vi "5 - filtering.vi"() -> ()   [LabVIEW 2025]
uses:
  <vilib>/Analysis/3filter.llb/Butterworth Filter (DBL).vi
  <vilib>/Waveform/WDTFileIO.llb/Export Waveform To Spreadsheet File.vi
  <vilib>/measure/NI_MABase.lvlib
  <vilib>/Analysis/NI_AALBase.lvlib
panel:
  in  "Sampling info":T1={"frequency [Hz]"=1000.0, "number of samples"=1000.0} {"number of samples" format="%.2p"; "frequency [Hz]" format="%.2p"}
  in  "time to refresh [ms]":u32
  in  "off/on":bool
  in  "off/on":bool
  in  "off/ on":bool
  out "filter characteristic":u16(ring) items=["Butterworth Filter", "Chebyshev Filter", "Elliptic Filter", "Bessel Filter"]
  in  "Tab Control":enum32{"waveform", "noise"}(tab)
  in  "phase [deg]":dbl(slide) scale=0.0..360.0
  in  "frequency [Hz]":dbl=10.0 min=0.0 format="%.0p"
  in  "offset [V]":dbl(slide) scale=0.0..10.0
  in  "amplitude [V]":dbl=1.0 min=0.0 format="%.0p"
  in  "signal type":u16(ring) items=["sine wave", "triangle wave", "square wave", "sawtooth wave"]
  in  "standard deviation":dbl=1.0 min=0.0 max=100.0 step=1.0 format="%.2f"
  in  "Tab Control":enum32{"waveform", "noise"}(tab)
  in  "frequency [Hz]":dbl=10.0 min=0.0 format="%.0p"
  in  "phase [deg]":dbl(slide) scale=0.0..360.0
  in  "offset [V]":dbl(slide) scale=0.0..10.0
  in  "amplitude [V]":dbl=1.0 min=0.0 format="%.0p"
  in  "signal type 2":u16(ring) items=["sine wave", "triangle wave", "square wave", "sawtooth wave"]
  in  "standard deviation":dbl=1.0 min=0.0 max=100.0 step=1.0 format="%.2f"
  in  "Tab Control":enum32{"waveform", "noise"}(tab)
  in  "phase [deg]":dbl(slide) scale=0.0..360.0
  in  "frequency [Hz]":dbl=10.0 min=0.0 format="%.0p"
  in  "offset [V]":dbl(slide) scale=0.0..10.0
  in  "amplitude [V]":dbl=1.0 min=0.0 format="%.0p"
  in  "signal type":u16(ring) items=["sine wave", "triangle wave", "square wave", "sawtooth wave"]
  in  "standard deviation":dbl=1.0 min=0.0 max=100.0 step=1.0 format="%.2f"
  in  "Tab Control":enum32{"Page 2"}(tab)
  in  "order":i32=2 min=0
  in  "high cutoff freq [Hz]":dbl=0.45000000000000007 min=0.0 format="%.1f"
  in  "filter type":u16(ring) items=["lowpass", "highpass", "bandpass", "bandstop"]
  in  "init/cont":bool
  in  "low cutoff freq [Hz]":dbl=0.12500000000000006 min=0.0 format="%.1f"
  out "Filter output":cluster{i32, dbl, "Filtered X":dbl[]}(graph)
  out "Filter input":waveform(dbl)(graph)
  in  "stop":bool
  # "Channel A"
  # "Channel B"
  # "Channel C"
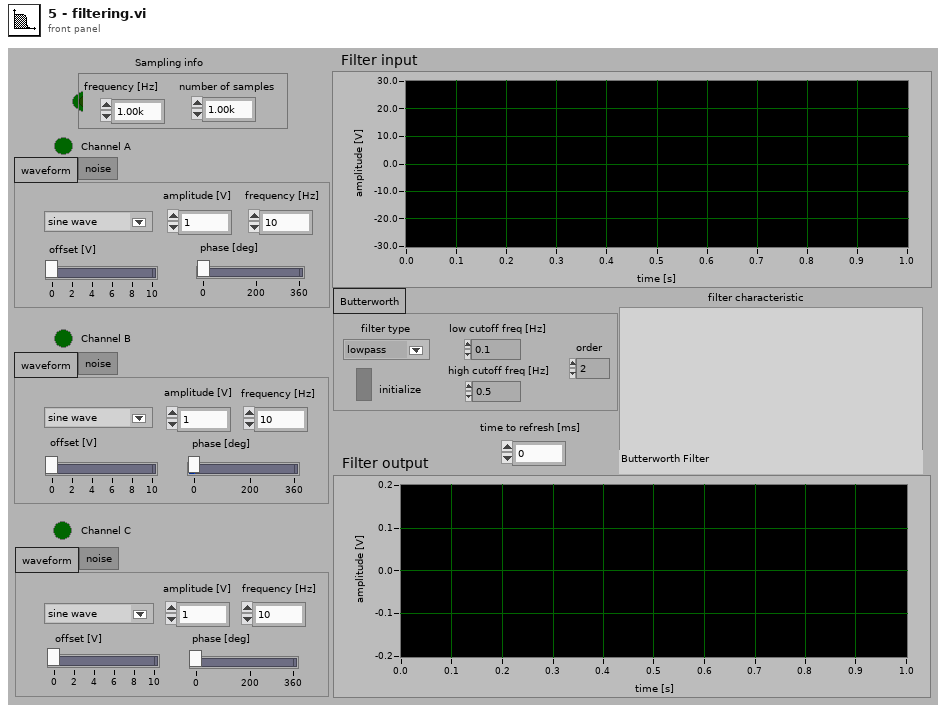
[diagram p1: front panel]
types:
  T1 = cluster{"frequency [Hz]":dbl, "number of samples":dbl}
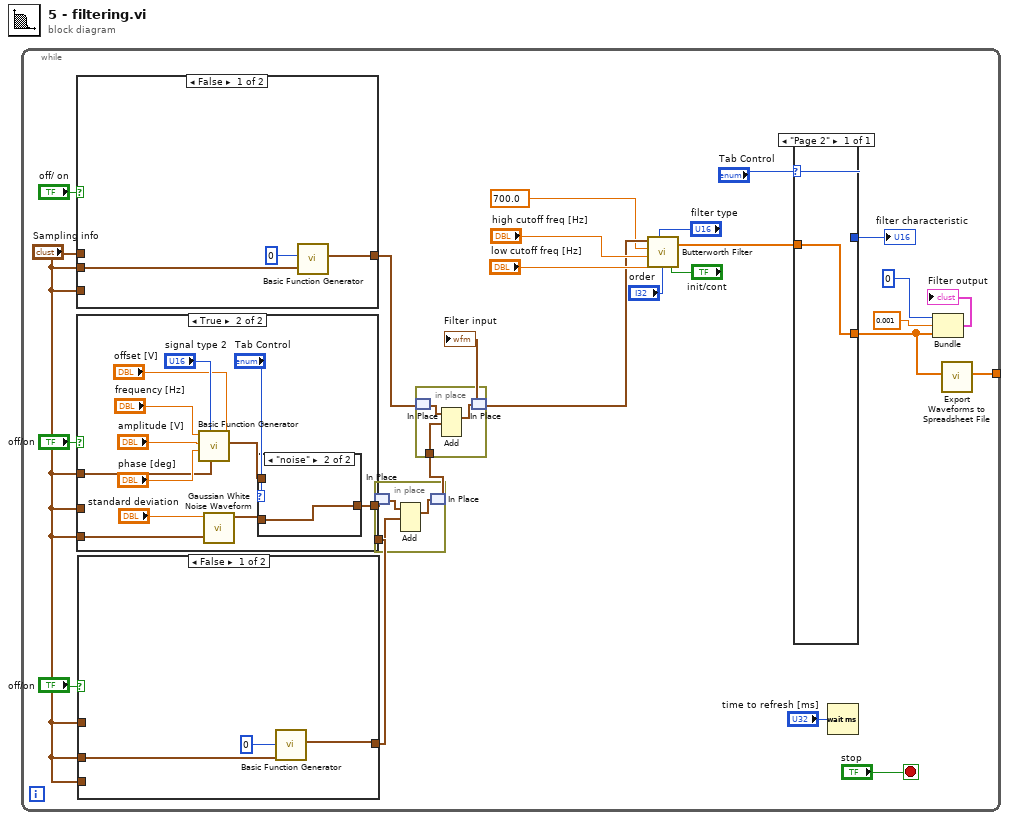
[diagram p0: block diagram]
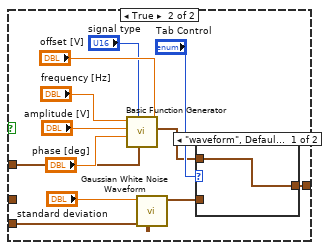
[diagram p2: hidden frame]
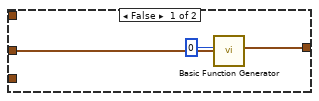
[diagram p4: hidden frame]
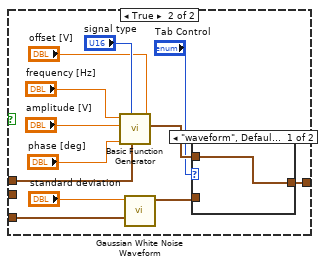
[diagram p6: hidden frame]
diagram:
  n1 = while {
    tunnel: [w6] -> w1
    stop <- "stop" stop-if-true
    n2 = case shown="False" "off/ on" {
      tunnel: [w68 w72] -> w5
      tunnel: "Sampling info" -> [_ w70]
      tunnel: "Sampling info" -> [_ w69]
      tunnel: "Sampling info" -> [w66 _]
      frame False {
        n3 = call <vilib>:"Basic Function Generator.vi"("sampling info"=w66, "amplitude"=0) -> ("signal out"=w68:waveform(dbl))  [unwired: 7 in, 2 out]
      }
      frame True {
        n4 = call <vilib>:"Basic Function Generator.vi"("offset"="offset [V]", "sampling info"=w69, "signal type"="signal type", "phase"="phase [deg]", "amplitude"="amplitude [V]", "frequency"="frequency [Hz]") -> ("signal out"=w80:waveform(dbl))  [unwired: 3 in, 2 out]
        n5 = call <vilib>:"Gaussian White Noise Waveform.vi"("sampling info"=w70, "standard deviation"="standard deviation") -> ("signal out"=w74:waveform(dbl))  [unwired: 3 in, 6 out]
        n6 = case shown="\"waveform\", Default" "Tab Control" {
          tunnel: w80 -> [w81 _]
          tunnel: w74 -> [_ w82]
          tunnel: [w81 w82] -> w72
          frame "waveform", Default {
          }
          frame "noise" {
          }
        }
      }
    }
    n7 = case shown="True" "off/on" {
      tunnel: [w50 w54] -> w21
      tunnel: "Sampling info" -> [_ w53]
      tunnel: "Sampling info" -> [_ w52]
      tunnel: "Sampling info" -> [w49 _]
      frame False {
        n8 = call <vilib>:"Basic Function Generator.vi"("sampling info"=w49, "amplitude"=0) -> ("signal out"=w50:waveform(dbl))  [unwired: 7 in, 2 out]
      }
      frame True {
        n9 = call <vilib>:"Basic Function Generator.vi"("offset"="offset [V]", "sampling info"=w52, "signal type"="signal type 2", "phase"="phase [deg]", "amplitude"="amplitude [V]", "frequency"="frequency [Hz]") -> ("signal out"=w63:waveform(dbl))  [unwired: 3 in, 2 out]
        n10 = call <vilib>:"Gaussian White Noise Waveform.vi"("sampling info"=w53, "standard deviation"="standard deviation") -> ("signal out"=w62:waveform(dbl))  [unwired: 3 in, 6 out]
        n11 = case shown="\"noise\"" "Tab Control" {
          tunnel: w63 -> [w64 _]
          tunnel: w62 -> [_ w65]
          tunnel: [w64 w65] -> w54
          frame "waveform", Default {
          }
          frame "noise" {
          }
        }
      }
    }
    n12 = case shown="False" "off/on" {
      tunnel: [w34 w45] -> w20
      tunnel: "Sampling info" -> [_ w36]
      tunnel: "Sampling info" -> [_ w35]
      tunnel: "Sampling info" -> [w32 _]
      frame False {
        n13 = call <vilib>:"Basic Function Generator.vi"("sampling info"=w32, "amplitude"=0) -> ("signal out"=w34:waveform(dbl))  [unwired: 7 in, 2 out]
      }
      frame True {
        n14 = call <vilib>:"Basic Function Generator.vi"("offset"="offset [V]", "sampling info"=w35, "signal type"="signal type", "phase"="phase [deg]", "amplitude"="amplitude [V]", "frequency"="frequency [Hz]") -> ("signal out"=w43:waveform(dbl))  [unwired: 3 in, 2 out]
        n15 = call <vilib>:"Gaussian White Noise Waveform.vi"("sampling info"=w36, "standard deviation"="standard deviation") -> ("signal out"=w46:waveform(dbl))  [unwired: 3 in, 6 out]
        n16 = case shown="\"waveform\", Default" "Tab Control" {
          tunnel: w43 -> [w47 _]
          tunnel: w46 -> [_ w48]
          tunnel: [w47 w48] -> w45
          frame "waveform", Default {
          }
          frame "noise" {
          }
        }
      }
    }
    n17 = in-place {
      in-place-border: w20 -> [w27]
      n18 = in-place-match #1(w21) -> (w28:waveform(dbl))
      n19 = Add ("Add Waveforms.vi")(1:w27, 2:w28) -> (0:w26:waveform(dbl))  [unwired: 1 in, 1 out]
      n20 = in-place-match #1(w26) -> (w19:waveform(dbl))
    }
    n21 = in-place {
      in-place-border: w19 -> [w31]
      n22 = in-place-match #2(w5) -> (w30:waveform(dbl))
      n23 = Add ("Add Waveforms.vi")(1:w31, 2:w30) -> (0:w29:waveform(dbl))  [unwired: 1 in, 1 out]
      n24 = in-place-match #2(w29) -> (w4:waveform(dbl))
    }
    "Filter input" <- w4
    n25 = call-poly <vilib>:"Butterworth Filter.vi"("init/cont (init:F)"="init/cont", "order"="order", "filter type"="filter type", "low cutoff freq: fl"="low cutoff freq [Hz]", "high cutoff freq: fh"="high cutoff freq [Hz]", "sampling freq: fs"=700.0, "X"=w4) -> ("Filtered X"=w11:dbl[])  [unwired: 2 out]
    n26 = case shown="\"Page 2\"" "Tab Control" {
      selector: "Tab Control" -> [w83]
      tunnel: w11 -> [w84]
      tunnel: [w84] -> w6
      tunnel: [w83] -> w12
      frame "Page 2" {
      }
    }
    "filter characteristic" <- w12
    n27 = Wait (ms)(milliseconds to wait="time to refresh [ms]") -> ()  [unwired: 1 out]
    n28 = Bundle(0, 0.001, "Filtered X"=w6) -> (→"Filter output":cluster{i32, dbl, "Filtered X":dbl[]})  [unwired: 1 out]
  }
  n29 = call-poly <vilib>:"Export Waveforms to Spreadsheet File.vi"("waveform"=w1) -> ()  [unwired: 6 in, 5 out]
